vi "nm to Percent Gate Width.vi"(0 "freq":dbl[unit], 1 "Gate Width":dbl[unit]) -> (4 "gatewidth%":dbl)   [LabVIEW 2023, in "Photon Counter.lvclass"]
uses:
  Photon Counter.lvclass
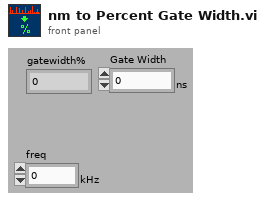
[diagram p1: front panel]
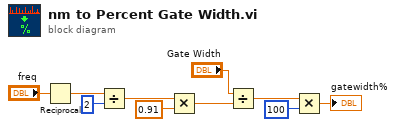
[diagram p0: block diagram]
diagram:
  n1 = Reciprocal(x="freq") -> (1/x=w1:dbl[unit])
  n2 = Divide(x=w1, y=2) -> (x/y=w9:dbl[unit])
  n3 = Multiply(x=w9, y=0.91) -> (x*y=w6:dbl[unit])
  n4 = Divide(x="Gate Width", y=w6) -> (x/y=w7:dbl)
  n5 = Multiply(x=w7, y=100) -> (x*y=→"gatewidth%":dbl)
